vi "readIVmode.vi"(7 "address":string, 8 "error in (no error)":errorcluster) -> (0 "error out":errorcluster, 3 "IV mode":T1)   [LabVIEW 2016]
doc: "API to get the results of lockin calculation.\n\nIf address=\"\", this API reads from localhost\nIf address is remote lockin, you need to add this computer to allowed whitelist on the lockin computer you are trying to access."
uses:
  RemoteControl/Typedefs/PrivateEvents--RemoteControl.setIVmode.ctl
  RemoteControl/Typedefs/Remote-SMO-Commands-Enum.ctl
  RemoteControl/RemoteControl.lvclass
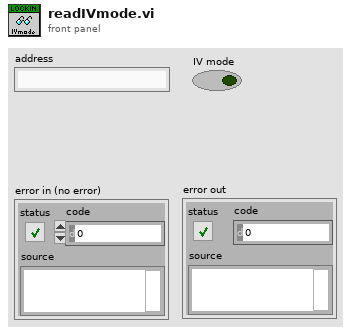
[diagram p1: front panel]
types:
  T1 = typedef "RemoteControl.lvclass/PrivateEvents--RemoteControl.setIVmode.ctl" = bool
  T2 = typedef "RemoteControl.lvclass/Remote-SMO-Commands-Enum.ctl" = enum16{"configAO", "configREF", "configIVmode", "configRemote", "configReset", "assertTrigger", "getAO", "getAI", "getResults", "getTrigger", "getIVmode", "getAOconfig", "getREFconfig", "ACK", "UNK", "CLOSE"}
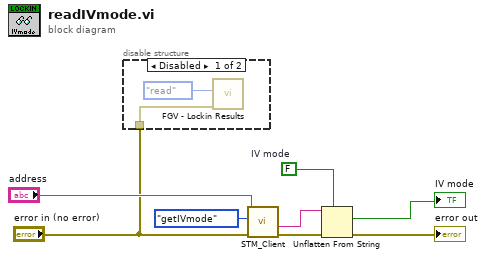
[diagram p0: block diagram]
diagram:
  w1 = T1 FALSE  # IV mode
  n1 = disable-structure shown="Disabled" {
    disable-tunnel: "error in (no error)" -> [w9 _]
    frame Disabled {
      n2 = call "FGV - Lockin Results.vi"("error in"=w9, "Function"=enum16{"write", "read"}."read") -> ()  [unwired: 4 in, 2 out]
    }
    frame Enabled {
    }
  }
  n3 = call "STM_Client.vi"("error in (no error)"="error in (no error)", "Command"=Remote-SMO-Commands-Enum."getIVmode", "address"="address") -> ("error out"=w7:errorcluster, "data received from server"=w3:string)  [unwired: 7 in]
  n4 = Unflatten From String(type=w1, binary string=w3, error in (no error)=w7) -> (value=→"IV mode":T1, error out=→"error out":errorcluster)  [unwired: 2 in, 1 out]
